vi "Convert to tiff.vi"(8 "error in (no error)":errorcluster, 9 "source file":path, 10 "Destination directory":path, 11 "reference to path":refnum<vi>) -> (0 "error out":errorcluster)   [LabVIEW 2012]
uses:
  DAQOrcaFlash/DAQOrcaFlash.lvclass
panel:
  out "Path":path
  out "Slide":sgl(slide) scale=0.0..1.0
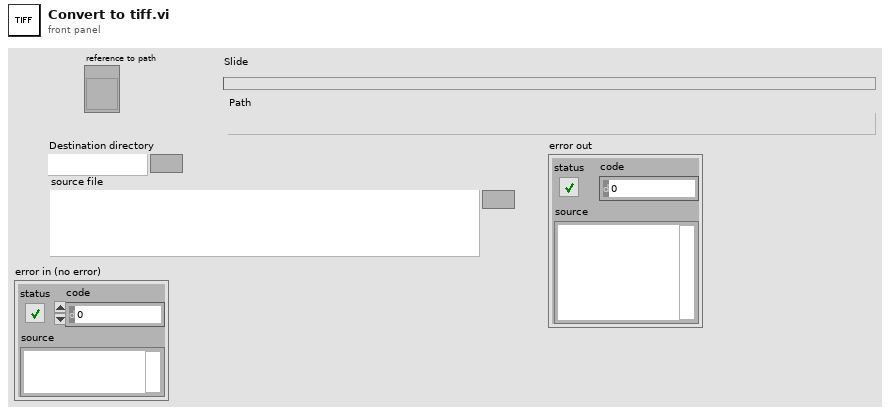
[diagram p1: front panel]
types:
  T1 = typedef "Image Type" = u32
  T2 = typedef "IMAQ Image.ctl" = refnum<image>
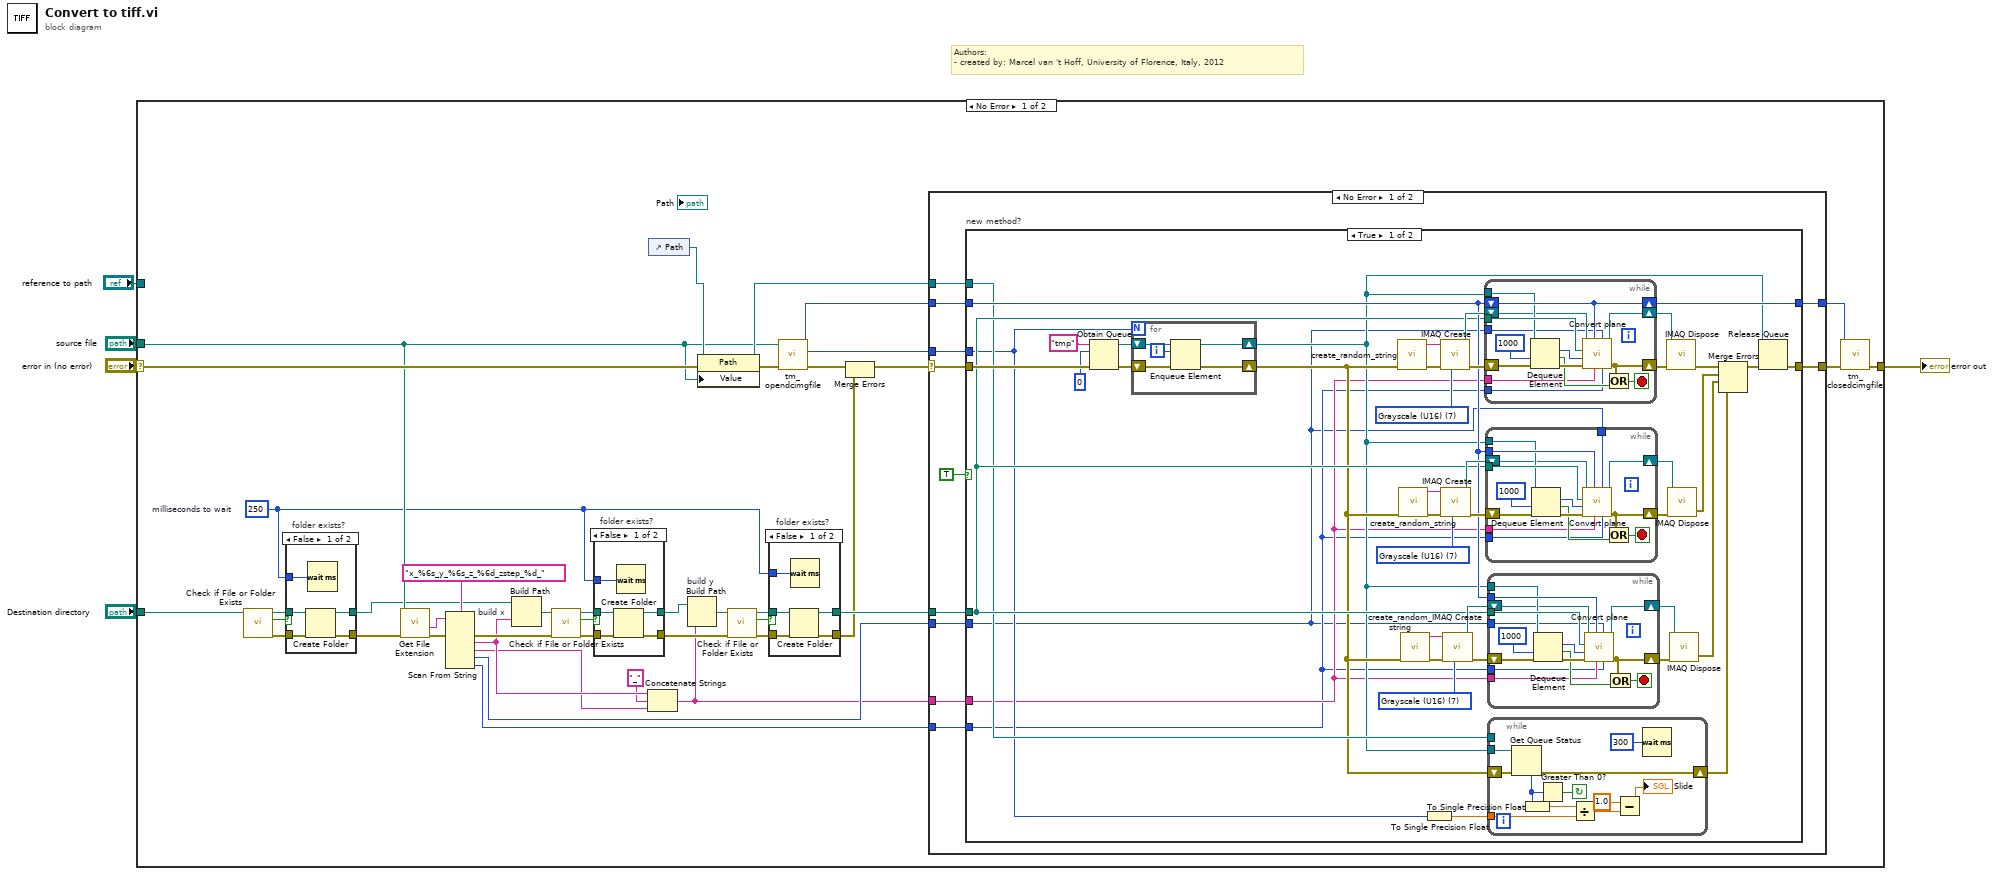
[diagram p0: block diagram]
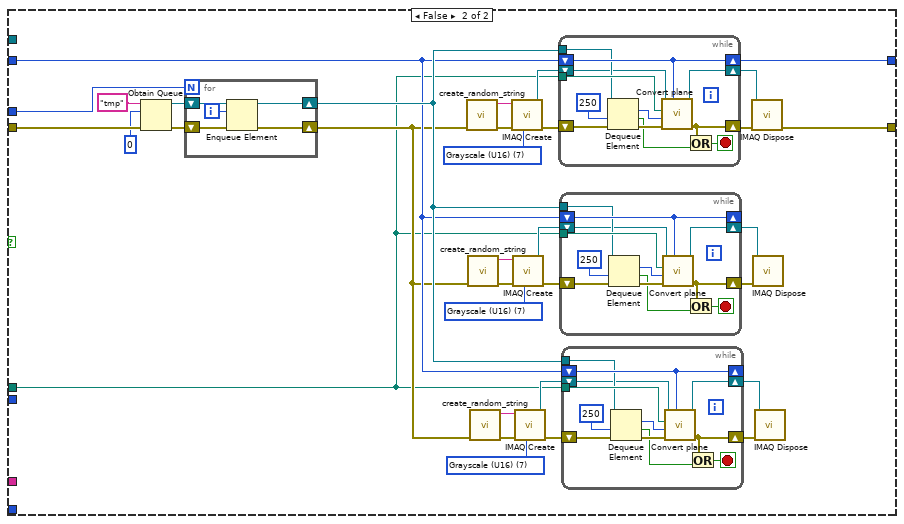
[diagram p5: hidden frame]
diagram:
  # "Authors: \n- created by: Marcel van 't Hoff, University of Florence, Italy, 2012"
  n1 = case shown="No Error" "error in (no error)" {
    selector: "error in (no error)" -> [w46 w259]
    tunnel: [w41 w259] -> w2
    tunnel: "source file" -> [w33 _]
    tunnel: "Destination directory" -> [w39 _]
    tunnel: "reference to path" -> [_ _]
    frame No Error {
      w6 = u32 250  # milliseconds to wait
      n2 = call <vilib>:"Check if File or Folder Exists.vi"("path"=w39) -> ("error out"=w36:errorcluster, "file or folder exists?"=w37:bool, "dup path"=w38:path)  [unwired: 8 in]
      n3 = case "folder exists?" shown="False" w37 {
        tunnel: [w65 w67] -> w16
        tunnel: w38 -> [w64 w67]
        tunnel: w36 -> [w63 w66]
        tunnel: [w62 w66] -> w29
        tunnel: w6 -> [w61 _]
        frame False {
          n4 = Create Folder(path (use dialog)=w64, error in=w63) -> (created path=w65:path, error out=w62:errorcluster)  [unwired: 1 in, 1 out]
          n5 = Wait (ms)(milliseconds to wait=w61) -> ()  [unwired: 1 out]
        }
        frame True {
        }
      }
      n6 = call <vilib>:"Get File Extension.vi"("error in (no error)"=w29, "file"=w33) -> ("error out"=w30:errorcluster, "filename without extension"=w31:string)  [unwired: 6 in, 2 out]
      n7 = Scan From String(format string="x_%6s_y_%6s_z_%6d_zstep_%d_", input string=w31, error in=w30) -> (error out=w25:errorcluster, output 1=w15:string, output 2=w13:string, output 3=w11:i32, output 4=w12:i32)  [unwired: 5 in, 2 out]
      n8 = Build Path "build x"(base path=w16, name or relative path=w15) -> (appended path=w24:path)
      n9 = call <vilib>:"Check if File or Folder Exists.vi"("error in (no error)"=w25, "path"=w24) -> ("error out"=w28:errorcluster, "file or folder exists?"=w27:bool, "dup path"=w26:path)  [unwired: 7 in]
      n10 = case "folder exists?" shown="False" w27 {
        tunnel: [w58 w60] -> w19
        tunnel: w26 -> [w57 w60]
        tunnel: w28 -> [w56 w59]
        tunnel: [w55 w59] -> w18
        tunnel: w6 -> [w54 _]
        frame False {
          n11 = Create Folder(path (use dialog)=w57, error in=w56) -> (created path=w58:path, error out=w55:errorcluster)  [unwired: 1 in, 1 out]
          n12 = Wait (ms)(milliseconds to wait=w54) -> ()  [unwired: 1 out]
        }
        frame True {
        }
      }
      n13 = Concatenate Strings(w15, "_" ("string"), w13) -> (w7:string)
      n14 = control-ref of="Path"() -> (w34:refnum<vi>)
      n15 = Build Path "build y"(base path=w19, name or relative path=w7) -> (appended path=w23:path)
      n16 = property class="Path"(reference=w34, error in=w46, "Value"=w33) -> (reference out=w35:refnum<vi>, error out=w40:errorcluster)
      n17 = call <vilib>:"Check if File or Folder Exists.vi"("error in (no error)"=w18, "path"=w23) -> ("error out"=w20:errorcluster, "file or folder exists?"=w21:bool, "dup path"=w22:path)  [unwired: 7 in]
      n18 = case "folder exists?" shown="False" w21 {
        tunnel: [w51 w53] -> w17
        tunnel: w22 -> [w50 w53]
        tunnel: w20 -> [w49 w52]
        tunnel: [w48 w52] -> w10
        tunnel: w6 -> [w47 _]
        frame False {
          n19 = Create Folder(path (use dialog)=w50, error in=w49) -> (created path=w51:path, error out=w48:errorcluster)  [unwired: 1 in, 1 out]
          n20 = Wait (ms)(milliseconds to wait=w47) -> ()  [unwired: 1 out]
        }
        frame True {
        }
      }
      n21 = call <userlib>:"tm_opendcimgfile.vi"("error in (no error)"=w40, "Path"=w33) -> ("error out"=w9:errorcluster, "Total Frames"=w45:i32, "File Handle"=w44:u32)  [unwired: 7 in]
      n22 = Merge Errors(w9, w10) -> (w8:errorcluster)
      n23 = case shown="No Error" w8 {
        selector: w8 -> [w78 w258]
        tunnel: w44 -> [w74 w257]
        tunnel: [w76 w258] -> w42
        tunnel: w45 -> [w75 _]
        tunnel: w17 -> [w73 _]
        tunnel: w35 -> [w71 _]
        tunnel: [w77 w257] -> w43
        tunnel: w7 -> [w70 _]
        tunnel: w12 -> [w69 _]
        tunnel: w11 -> [w68 _]
        frame No Error {
          n24 = case "new method?" shown="True" TRUE {
            tunnel: w78 -> [w115 w209]
            tunnel: [w114 w208] -> w77
            tunnel: [w83 w207] -> w76
            tunnel: w75 -> [w90 w200]
            tunnel: w74 -> [w98 w189]
            tunnel: w73 -> [w97 w187]
            tunnel: w71 -> [w92 _]
            tunnel: w70 -> [w81 _]
            tunnel: w69 -> [w80 _]
            tunnel: w68 -> [w79 _]
            frame True {
              w100 = T1 7 items=["Grayscale (U8)", "Grayscale (I16)", "Grayscale (SGL)", "Complex (CSG)", "RGB (U32)", "HSL (U32)", "RGB (U64)", "Grayscale (U16)"] ("Image Type")
              w112 = T1 7 items=["Grayscale (U8)", "Grayscale (I16)", "Grayscale (SGL)", "Complex (CSG)", "RGB (U32)", "HSL (U32)", "RGB (U64)", "Grayscale (U16)"] ("Image Type")
              w117 = T1 7 items=["Grayscale (U8)", "Grayscale (I16)", "Grayscale (SGL)", "Complex (CSG)", "RGB (U32)", "HSL (U32)", "RGB (U64)", "Grayscale (U16)"] ("Image Type")
              n25 = Obtain Queue(name (unnamed)="tmp", element data type=0, error in (no error)=w115) -> (queue out=w93:refnum<queue>, error out=w96:errorcluster)  [unwired: 2 in, 1 out]
              n26 = for {
                N: w90 -> [_]
                shift-right: [w134] -> w91
                shift-left: w96 -> [w137]
                shift-right: [w133] -> w82
                shift-left: w93 -> [w136]
                i -> [w135]
                n27 = Enqueue Element(queue=w136, element=w135, error in (no error)=w137) -> (queue out=w133:refnum<queue>, error out=w134:errorcluster)  [unwired: 1 in, 1 out]
              }
              n28 = call "create_random_string.vi"("error in (no error)"=w91) -> ("error out"=w119:errorcluster, "random string"=w118:string)  [unwired: 9 in]
              n29 = call "create_random_string.vi"("error in (no error)"=w91) -> ("error out"=w110:errorcluster, "random string"=w111:string)  [unwired: 9 in]
              n30 = call "create_random_string.vi"("error in (no error)"=w91) -> ("error out"=w102:errorcluster, "random string"=w101:string)  [unwired: 9 in]
              n31 = To Single Precision Float(number=w90) -> (single precision float=w89:sgl)
              n32 = call "IMAQ Create"("Image Name"=w118, "Image Type"=w117, "error in (no error)"=w119) -> ("New Image"=w120:T2, "error out"=w116:errorcluster)  [unwired: 2 in]
              n33 = call "IMAQ Create"("Image Name"=w111, "Image Type"=w112, "error in (no error)"=w110) -> ("New Image"=w109:T2, "error out"=w113:errorcluster)  [unwired: 2 in]
              n34 = call "IMAQ Create"("Image Name"=w101, "Image Type"=w100, "error in (no error)"=w102) -> ("New Image"=w103:T2, "error out"=w99:errorcluster)  [unwired: 2 in]
              n35 = while {
                tunnel: w97 -> [w182]
                shift-right: [w173] -> w107
                shift-left: w116 -> [w178]
                shift-right: [w181] -> w121
                shift-left: w120 -> [w176]
                shift-right: [w180] -> w114
                shift-left: w98 -> [w180]
                tunnel: w82 -> [w179]
                tunnel: w81 -> [w170]
                tunnel: w80 -> [w169]
                tunnel: w79 -> [w168]
                stop <- w171 stop-if-true
                n36 = Dequeue Element(queue=w179, timeout in ms (-1)=1000, error in (no error)=w178) -> (element=w177:i32, timed out?=w172:bool, error out=w174:errorcluster)  [unwired: 1 out]
                n37 = call "Convert plane.vi"("z step size"=w169, "z start position"=w168, "basepath name"=w170, "File Handle"=w180, "error in (no error)"=w174, "Frame Index"=w177, "file in"=w182, "Image in"=w176) -> ("error out"=w173:errorcluster, "Image out"=w181:T2)  [unwired: 2 in]
                n38 = Or(x=w173, y=w172) -> (x .or. y?=w171:bool)
              }
              n39 = while {
                tunnel: w97 -> [w167]
                shift-right: [w156] -> w106
                shift-left: w113 -> [w163]
                shift-right: [w166] -> w108
                shift-left: w109 -> [w160]
                tunnel: w82 -> [w164]
                tunnel: w98 -> [w165]
                tunnel: w81 -> [w155]
                tunnel: w80 -> [w154]
                tunnel: w79 -> [w153]
                stop <- w157 stop-if-true
                n40 = Dequeue Element(queue=w164, timeout in ms (-1)=1000, error in (no error)=w163) -> (element=w161:i32, timed out?=w158:bool, error out=w162:errorcluster)  [unwired: 1 out]
                n41 = call "Convert plane.vi"("z step size"=w154, "z start position"=w153, "basepath name"=w155, "File Handle"=w165, "error in (no error)"=w162, "Frame Index"=w161, "file in"=w167, "Image in"=w160) -> ("error out"=w156:errorcluster, "Image out"=w166:T2)  [unwired: 2 in]
                n42 = Or(x=w156, y=w158) -> (x .or. y?=w157:bool)
              }
              n43 = while {
                tunnel: w97 -> [w152]
                shift-right: [w141] -> w105
                shift-left: w99 -> [w148]
                shift-right: [w151] -> w104
                shift-left: w103 -> [w145]
                tunnel: w82 -> [w149]
                tunnel: w98 -> [w150]
                tunnel: w81 -> [w140]
                tunnel: w80 -> [w139]
                tunnel: w79 -> [w138]
                stop <- w142 stop-if-true
                n44 = Dequeue Element(queue=w149, timeout in ms (-1)=1000, error in (no error)=w148) -> (element=w146:i32, timed out?=w143:bool, error out=w147:errorcluster)  [unwired: 1 out]
                n45 = call "Convert plane.vi"("z step size"=w139, "z start position"=w138, "basepath name"=w140, "File Handle"=w150, "error in (no error)"=w147, "Frame Index"=w146, "file in"=w152, "Image in"=w145) -> ("error out"=w141:errorcluster, "Image out"=w151:T2)  [unwired: 2 in]
                n46 = Or(x=w141, y=w143) -> (x .or. y?=w142:bool)
              }
              n47 = while {
                tunnel: w82 -> [w132]
                tunnel: w92 -> [_]
                shift-right: [w123] -> w86
                shift-left: w91 -> [w130]
                tunnel: w89 -> [w128]
                stop <- w131 continue-if-true
                n48 = Get Queue Status(queue=w132, error in (no error)=w130) -> (error out=w123:errorcluster, # elements in queue=w129:i32)  [unwired: 1 in, 6 out]
                n49 = To Single Precision Float(number=w129) -> (single precision float=w127:sgl)
                n50 = Greater Than 0?(x=w129) -> (x > 0?=w131:bool)
                n51 = Divide(x=w127, y=w128) -> (x/y=w125:sgl)
                n52 = Subtract(x=sgl 1.0, y=w125) -> (x-y=→"Slide":sgl)
                n53 = Wait (ms)(milliseconds to wait=u32 300) -> ()  [unwired: 1 out]
              }
              n54 = call "IMAQ Dispose"("Image"=w121, "error in (no error)"=w107) -> ("error out"=w85:errorcluster)  [unwired: 4 in]
              n55 = call "IMAQ Dispose"("Image"=w108, "error in (no error)"=w106) -> ("error out"=w88:errorcluster)  [unwired: 4 in]
              n56 = call "IMAQ Dispose"("Image"=w104, "error in (no error)"=w105) -> ("error out"=w87:errorcluster)  [unwired: 4 in]
              n57 = Merge Errors(w85, w88, w87, w86) -> (w84:errorcluster)
              n58 = Release Queue(queue=w82, error in (no error)=w84) -> (error out=w83:errorcluster)  [unwired: 1 in, 2 out]
            }
            frame False {
              w192 = T1 7 items=["Grayscale (U8)", "Grayscale (I16)", "Grayscale (SGL)", "Complex (CSG)", "RGB (U32)", "HSL (U32)", "RGB (U64)", "Grayscale (U16)"] ("Image Type")
              w205 = T1 7 items=["Grayscale (U8)", "Grayscale (I16)", "Grayscale (SGL)", "Complex (CSG)", "RGB (U32)", "HSL (U32)", "RGB (U64)", "Grayscale (U16)"] ("Image Type")
              w211 = T1 7 items=["Grayscale (U8)", "Grayscale (I16)", "Grayscale (SGL)", "Complex (CSG)", "RGB (U32)", "HSL (U32)", "RGB (U64)", "Grayscale (U16)"] ("Image Type")
              n59 = Obtain Queue(name (unnamed)="tmp", element data type=0, error in (no error)=w209) -> (queue out=w183:refnum<queue>, error out=w186:errorcluster)  [unwired: 2 in, 1 out]
              n60 = for {
                N: w200 -> [_]
                shift-right: [w217] -> w188
                shift-left: w186 -> [w220]
                shift-right: [w216] -> w190
                shift-left: w183 -> [w219]
                i -> [w218]
                n61 = Enqueue Element(queue=w219, element=w218, error in (no error)=w220) -> (queue out=w216:refnum<queue>, error out=w217:errorcluster)  [unwired: 1 in, 1 out]
              }
              n62 = call "create_random_string.vi"("error in (no error)"=w188) -> ("error out"=w213:errorcluster, "random string"=w212:string)  [unwired: 9 in]
              n63 = call "create_random_string.vi"("error in (no error)"=w188) -> ("error out"=w203:errorcluster, "random string"=w204:string)  [unwired: 9 in]
              n64 = call "create_random_string.vi"("error in (no error)"=w188) -> ("error out"=w194:errorcluster, "random string"=w193:string)  [unwired: 9 in]
              n65 = call "IMAQ Create"("Image Name"=w212, "Image Type"=w211, "error in (no error)"=w213) -> ("New Image"=w214:T2, "error out"=w210:errorcluster)  [unwired: 2 in]
              n66 = call "IMAQ Create"("Image Name"=w204, "Image Type"=w205, "error in (no error)"=w203) -> ("New Image"=w202:T2, "error out"=w206:errorcluster)  [unwired: 2 in]
              n67 = call "IMAQ Create"("Image Name"=w193, "Image Type"=w192, "error in (no error)"=w194) -> ("New Image"=w195:T2, "error out"=w191:errorcluster)  [unwired: 2 in]
              n68 = while {
                tunnel: w187 -> [w256]
                shift-right: [w247] -> w199
                shift-left: w210 -> [w252]
                shift-right: [w255] -> w215
                shift-left: w214 -> [w250]
                shift-right: [w254] -> w208
                shift-left: w189 -> [w254]
                tunnel: w190 -> [w253]
                stop <- w245 stop-if-true
                n69 = Dequeue Element(queue=w253, timeout in ms (-1)=250, error in (no error)=w252) -> (element=w251:i32, timed out?=w246:bool, error out=w248:errorcluster)  [unwired: 1 out]
                n70 = call "Convert plane.vi"("File Handle"=w254, "error in (no error)"=w248, "Frame Index"=w251, "file in"=w256, "Image in"=w250) -> ("error out"=w247:errorcluster, "Image out"=w255:T2)  [unwired: 5 in]
                n71 = Or(x=w247, y=w246) -> (x .or. y?=w245:bool)
              }
              n72 = while {
                tunnel: w187 -> [w244]
                shift-right: [w233] -> w198
                shift-left: w206 -> [w240]
                shift-right: [w243] -> w201
                shift-left: w202 -> [w237]
                shift-right: [w242] -> _
                shift-left: w189 -> [w242]
                tunnel: w190 -> [w241]
                stop <- w234 stop-if-true
                n73 = Dequeue Element(queue=w241, timeout in ms (-1)=250, error in (no error)=w240) -> (element=w238:i32, timed out?=w235:bool, error out=w239:errorcluster)  [unwired: 1 out]
                n74 = call "Convert plane.vi"("File Handle"=w242, "error in (no error)"=w239, "Frame Index"=w238, "file in"=w244, "Image in"=w237) -> ("error out"=w233:errorcluster, "Image out"=w243:T2)  [unwired: 5 in]
                n75 = Or(x=w233, y=w235) -> (x .or. y?=w234:bool)
              }
              n76 = while {
                tunnel: w187 -> [w232]
                shift-right: [w221] -> w197
                shift-left: w191 -> [w228]
                shift-right: [w231] -> w196
                shift-left: w195 -> [w225]
                shift-right: [w230] -> _
                shift-left: w189 -> [w230]
                tunnel: w190 -> [w229]
                stop <- w222 stop-if-true
                n77 = Dequeue Element(queue=w229, timeout in ms (-1)=250, error in (no error)=w228) -> (element=w226:i32, timed out?=w223:bool, error out=w227:errorcluster)  [unwired: 1 out]
                n78 = call "Convert plane.vi"("File Handle"=w230, "error in (no error)"=w227, "Frame Index"=w226, "file in"=w232, "Image in"=w225) -> ("error out"=w221:errorcluster, "Image out"=w231:T2)  [unwired: 5 in]
                n79 = Or(x=w221, y=w223) -> (x .or. y?=w222:bool)
              }
              n80 = call "IMAQ Dispose"("Image"=w215, "error in (no error)"=w199) -> ("error out"=w207:errorcluster)  [unwired: 4 in]
              n81 = call "IMAQ Dispose"("Image"=w201, "error in (no error)"=w198) -> ()  [unwired: 4 in, 1 out]
              n82 = call "IMAQ Dispose"("Image"=w196, "error in (no error)"=w197) -> ()  [unwired: 4 in, 1 out]
            }
          }
        }
        frame Error {
        }
      }
      n83 = call <userlib>:"tm_closedcimgfile.vi"("error in (no error)"=w42, "File Handle"=w43) -> ("error out"=w41:errorcluster)  [unwired: 9 in]
    }
    frame Error {
    }
  }
  "error out" <- w2
